vi "波形图表上下限特色显示及绝对时间.vi"() -> ()   [LabVIEW 2017]
panel:
  in  "延时":u32=10
  in  "下限":dbl(slide)=-0.5592417061611374
  in  "上限":dbl(slide)=0.5639810426540285 scale=0.0..1.0
  out "波形图表":T1(graph)={"上限"=0.5639810426540285, "number: 0 to 1"=nan, "number: 0 to 1"=-0.7880107536067218, "下限"=-0.5592417061611374}
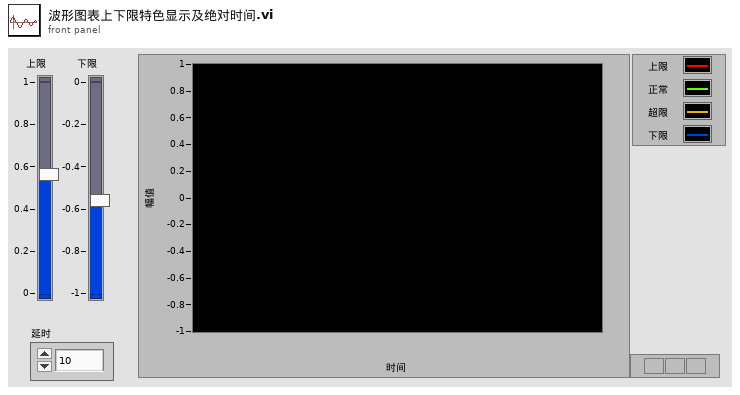
[diagram p1: front panel]
types:
  T1 = cluster{"上限":dbl, "number: 0 to 1":dbl, "number: 0 to 1":dbl, "下限":dbl}
  T2 = cluster{"上限":dbl, "number: 0 to 1":dbl, "number: 0 to 1":dbl, "下限":dbl}[]
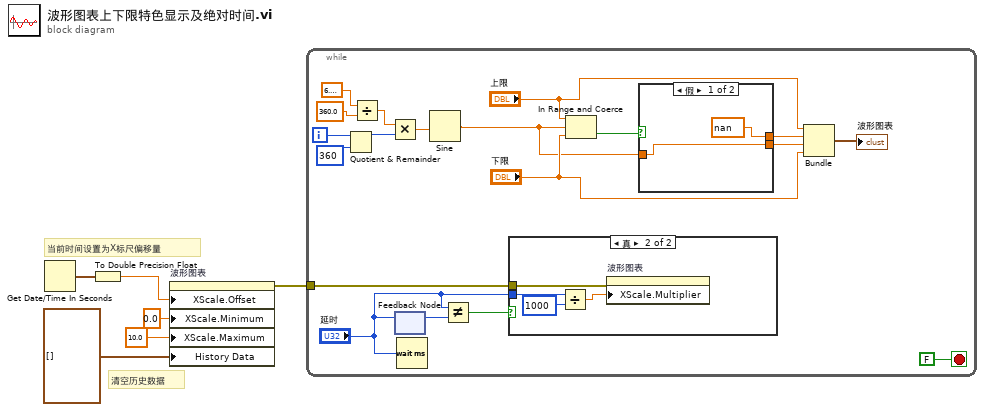
[diagram p0: block diagram]
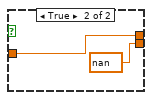
[diagram p3: hidden frame]
diagram:
  # "清空历史数据"
  # "当前时间设置为X标尺偏移量"
  n1 = Get Date/Time In Seconds() -> (seconds since 1Jan1904=w1:timestamp)
  n2 = To Double Precision Float(number=w1) -> (double precision float=w2:dbl)
  n3 = property on="波形图表" class="WFChart (严格)"("XScale.Offset"=w2, "XScale.Minimum"=0.0 ("X标尺.范围:最小值"), "XScale.Maximum"=10.0 ("X标尺.范围:最大值"), "History Data"=T2 [] ("历史数据")) -> (error out=w6:errorcluster)  [unwired: 2 in, 1 out]
  n4 = while {
    tunnel: w6 -> [w7]
    i -> [w17]
    stop <- FALSE stop-if-true
    n5 = Quotient & Remainder(x=w17, y=360) -> (x-y*floor(x/y)=w14:i32)  [unwired: 1 out]
    n6 = Divide(x=6.283185307179586, y=360.0) -> (x/y=w12:dbl)
    n7 = Multiply(x=w12, y=w14) -> (x*y=w15:dbl)
    n8 = feedback-in #1("延时") -> ()
    n9 = feedback #1() -> (w10:u32)  [unwired: 1 in]
    n10 = Wait (ms)(milliseconds to wait="延时") -> ()  [unwired: 1 out]
    n11 = Sine(x=w15) -> (sin(x)=w18:dbl)
    n12 = Not Equal?(x="延时", y=w10) -> (x != y?=w9:bool)
    n13 = case shown="真" w9 {
      tunnel: "延时" -> [_ w29]
      tunnel: w7 -> [_ w28]
      frame False {
      }
      frame True {
        n14 = Divide(x=w29, y=u32 1000) -> (x/y=w27:dbl)
        n15 = property on="波形图表" class="WFChart (严格)"(error in=w28, "XScale.Multiplier"=w27) -> ()  [unwired: 1 in, 2 out]
      }
    }
    n16 = In Range and Coerce(upper limit="上限", x=w18, lower limit="下限") -> (In Range?=w24:bool)  [unwired: 1 out]
    n17 = case shown="假" w24 {
      tunnel: w18 -> [w30 w32]
      tunnel: [w30 nan] -> w21
      tunnel: [nan w32] -> w20
      frame False {
      }
      frame True {
      }
    }
    n18 = Bundle("上限"="上限", w20, w21, "下限"="下限") -> (→"波形图表":cluster{"上限":dbl, dbl, dbl, "下限":dbl})  [unwired: 1 in]
  }
